vi "Redo.vi"(7 "Map Model in":refnum<class "Map Model.lvclass">, 8 "error in (no error)":errorcluster, 11 "Pan in":refnum<class "Pan.lvclass">) -> (0 "error out":errorcluster, 3 "Pan out":refnum<class "Pan.lvclass">, 5 "Map Model out":refnum<class "Map Model.lvclass">)   [LabVIEW 2020, in "Map Model.lvlib" / "Pan.lvclass"]
uses:
  Pan.lvclass
  E:/Project/Labview-Projects/Completed projects/Map Editor/Models/Map Model/Tools/Tool/Tool.lvclass
  Map Model/Map Model.lvclass
  Map Model/Map Model.lvclass/Map Model.ctl
  Tool/Tool.lvclass/Tool.ctl
  Tool/Tool.lvclass
panel:
  # "NOTICE -- YOU MUST LEAVE THIS NOTICE IN PLACE.\n\nCopyright (c) 2017, LIANG LIU Shawn.Liu.cn@gmail.com\nAll rights reserved.\n\nRedistribution and use in source and binary forms, with or without modification, are permitted provided that the following conditions are met:\n-Redistributions of source code must retain the above copyright notice, this list of conditions and the following disclaimer.\n-Redistributions in binary form must reproduce the above copyright notice, this list of conditions and the following disclaimer in the documentation and/or other materials provided with the distribution.\n-Neither the name of the eLp nor the names of its contributors may be used to endorse or promote products derived from this software without specific prior written permission.\n\nTHIS SOFTWARE IS PROVIDED BY THE COPYRIGHT HOLDERS AND CONTRIBUTORS \"AS IS\" AND ANY EXPRESS OR IMPLIED WARRANTIES, INCLUDING, BUT NOT LIMITED TO, THE IMPLIED WARRANTIES OF MERCHANTABILITY AND FITNESS FOR A PARTICULAR PURPOSE ARE DISCLAIMED. IN NO EVENT SHALL THE COPYRIGHT HOLDER OR CONTRIBUTORS BE LIABLE FOR ANY DIRECT, INDIRECT, INCIDENTAL, SPECIAL, EXEMPLARY, OR CONSEQUENTIAL DAMAGES (INCLUDING, BUT NOT LIMITED TO, PROCUREMENT OF SUBSTITUTE GOODS OR SERVICES; LOSS OF USE, DATA, OR PROFITS; OR BUSINESS INTERRUPTION) HOWEVER CAUSED AND ON ANY THEORY OF LIABILITY, WHETHER IN CONTRACT, STRICT LIABILITY, OR TORT (INCLUDING NEGLIGENCE OR OTHERWISE) ARISING IN ANY WAY OUT OF THE USE OF THIS SOFTWARE, EVEN IF ADVISED OF THE POSSIBILITY OF SUCH DAMAGE."
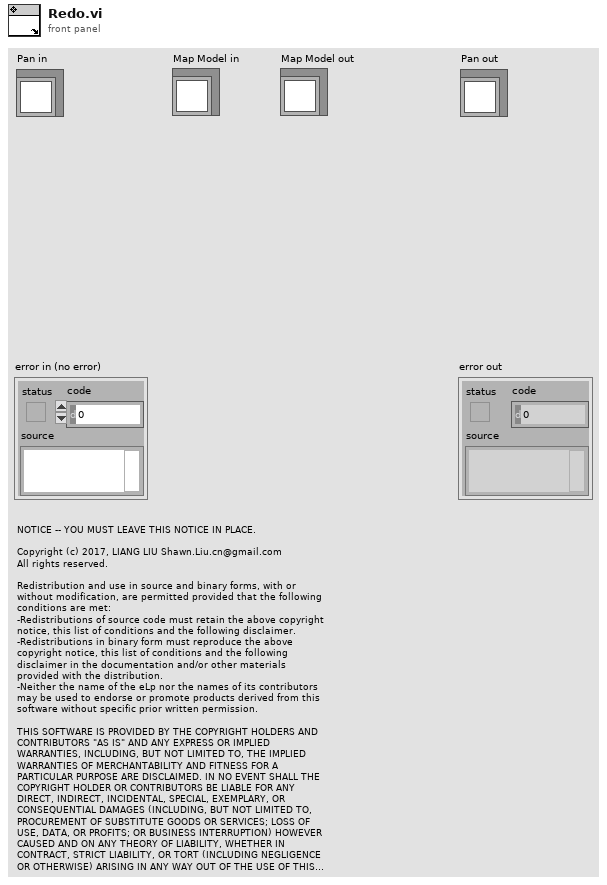
[diagram p1: front panel]
types:
  T1 = typedef "LVPoint32TypeDef.ctl" = cluster{"Horizontal":i32, "Vertical":i32}
  T2 = typedef "LVPointTypeDef.ctl" = cluster{"Horizontal":i16, "Vertical":i16}
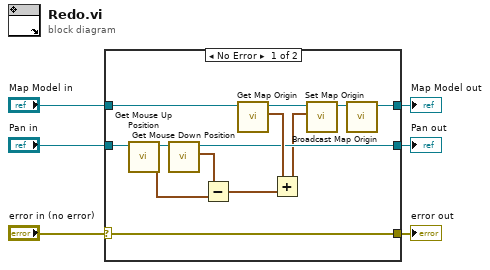
[diagram p0: block diagram]
diagram:
  n1 = case shown="No Error" "error in (no error)" {
    selector: "error in (no error)" -> [w8 w22]
    tunnel: "Map Model in" -> [w14 w21]
    tunnel: "Pan in" -> [w13 w20]
    tunnel: [w11 w20] -> w3
    tunnel: [w10 w21] -> w4
    tunnel: [w8 w22] -> w2
    frame No Error {
      n2 = call "Get Mouse Up Position.vi"("Tool in"=w13) -> ("Mouse Up Position"=w9:T1, "Tool out"=w12:refnum<class "Pan.lvclass">)  [unwired: 9 in]
      n3 = call "Get Mouse Down Position.vi"("Tool in"=w12) -> ("Mouse Down Position"=w19:T1, "Tool out"=w11:refnum<class "Pan.lvclass">)  [unwired: 9 in]
      n4 = Subtract(x=w19, y=w9) -> (x-y=w15:T1)
      n5 = call "Get Map Origin.vi"("Map Model in"=w14) -> ("Map Origin"=w16:T2, "Map Model out"=w18:refnum<class "Map Model.lvclass">)  [unwired: 9 in]
      n6 = Add(x=w16, y=w15) -> (x+y=w7:T1)
      n7 = call "Set Map Origin.vi"("Map Origin"=w7, "Map Model in"=w18) -> ("Map Model out"=w17:refnum<class "Map Model.lvclass">)  [unwired: 9 in]
      n8 = call "Broadcast Map Origin.vi"("Map Model in"=w17) -> ("Map Model out"=w10:refnum<class "Map Model.lvclass">)  [unwired: 9 in, 1 out]
    }
    frame Error {
    }
  }
  "error out" <- w2
  "Pan out" <- w3
  "Map Model out" <- w4
